vi "PI_12.vi"(7 "SLMAX":fxp<+/-,18,5>, 10 "ziyi_f_in":T1=[0.0, 0.0, 0.0, 0.0, 0.0, 0.0, 0.0, 0.0, 0.0, 0.0, 0.0, 0.0]) -> (2 "ziyi_f_out":T1)   [LabVIEW 2017]
uses:
  ziyi_pipe.ctl
  x_qp_scalar.ctl
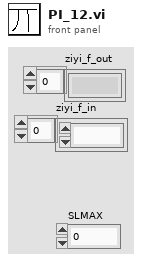
[diagram p1: front panel]
types:
  T1 = typedef "ziyi_pipe.ctl" = T2[]
  T2 = typedef "x_qp_scalar.ctl" = fxp<+/-,32,6>
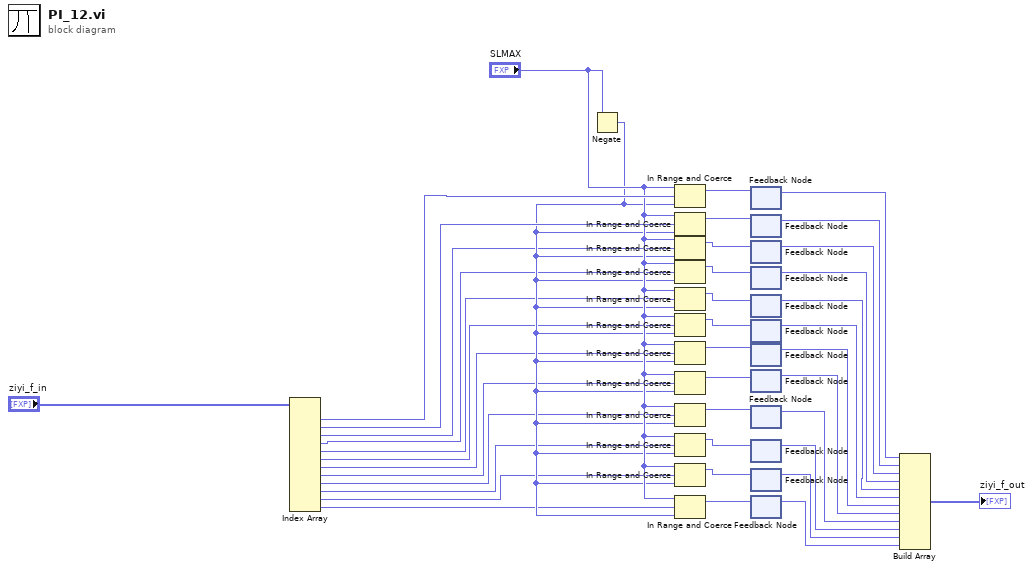
[diagram p0: block diagram]
diagram:
  n1 = Index Array(array="ziyi_f_in") -> (element #1=w16:T2, element #2=w15:T2, element #3=w12:T2, element #4=w11:T2, element #5=w10:T2, element #6=w9:T2, element #7=w8:T2, element #8=w7:T2, element #9=w6:T2, element #10=w5:T2, element #11=w4:T2, element #12=w3:T2)  [unwired: 12 in]
  n2 = Negate(x="SLMAX") -> (-x=w13:fxp<+/-,18,4>)
  n3 = In Range and Coerce(upper limit="SLMAX", x=w16, lower limit=w13) -> (coerced(x)=w40:T2)  [unwired: 1 out]
  n4 = In Range and Coerce(upper limit="SLMAX", x=w15, lower limit=w13) -> (coerced(x)=w39:T2)  [unwired: 1 out]
  n5 = In Range and Coerce(upper limit="SLMAX", x=w12, lower limit=w13) -> (coerced(x)=w38:T2)  [unwired: 1 out]
  n6 = In Range and Coerce(upper limit="SLMAX", x=w11, lower limit=w13) -> (coerced(x)=w37:T2)  [unwired: 1 out]
  n7 = In Range and Coerce(upper limit="SLMAX", x=w10, lower limit=w13) -> (coerced(x)=w36:T2)  [unwired: 1 out]
  n8 = In Range and Coerce(upper limit="SLMAX", x=w9, lower limit=w13) -> (coerced(x)=w35:T2)  [unwired: 1 out]
  n9 = In Range and Coerce(upper limit="SLMAX", x=w8, lower limit=w13) -> (coerced(x)=w34:T2)  [unwired: 1 out]
  n10 = In Range and Coerce(upper limit="SLMAX", x=w7, lower limit=w13) -> (coerced(x)=w33:T2)  [unwired: 1 out]
  n11 = In Range and Coerce(upper limit="SLMAX", x=w6, lower limit=w13) -> (coerced(x)=w32:T2)  [unwired: 1 out]
  n12 = In Range and Coerce(upper limit="SLMAX", x=w5, lower limit=w13) -> (coerced(x)=w31:T2)  [unwired: 1 out]
  n13 = In Range and Coerce(upper limit="SLMAX", x=w4, lower limit=w13) -> (coerced(x)=w30:T2)  [unwired: 1 out]
  n14 = In Range and Coerce(upper limit="SLMAX", x=w3, lower limit=w13) -> (coerced(x)=w29:T2)  [unwired: 1 out]
  n15 = feedback #1() -> (w28:T2)  [unwired: 1 in]
  n16 = feedback-in #1(w40) -> ()
  n17 = feedback #2() -> (w27:T2)  [unwired: 1 in]
  n18 = feedback-in #2(w39) -> ()
  n19 = feedback #3() -> (w26:T2)  [unwired: 1 in]
  n20 = feedback-in #3(w38) -> ()
  n21 = feedback #4() -> (w25:T2)  [unwired: 1 in]
  n22 = feedback-in #4(w37) -> ()
  n23 = feedback #5() -> (w24:T2)  [unwired: 1 in]
  n24 = feedback-in #5(w36) -> ()
  n25 = feedback #6() -> (w23:T2)  [unwired: 1 in]
  n26 = feedback-in #6(w35) -> ()
  n27 = feedback #7() -> (w22:T2)  [unwired: 1 in]
  n28 = feedback-in #7(w34) -> ()
  n29 = feedback #8() -> (w21:T2)  [unwired: 1 in]
  n30 = feedback-in #8(w33) -> ()
  n31 = feedback #9() -> (w20:T2)  [unwired: 1 in]
  n32 = feedback-in #9(w32) -> ()
  n33 = feedback #10() -> (w19:T2)  [unwired: 1 in]
  n34 = feedback-in #10(w31) -> ()
  n35 = feedback #11() -> (w18:T2)  [unwired: 1 in]
  n36 = feedback-in #11(w30) -> ()
  n37 = feedback #12() -> (w17:T2)  [unwired: 1 in]
  n38 = feedback-in #12(w29) -> ()
  n39 = Build Array(w28, w27, w26, w25, w24, w23, w22, w21, w20, w19, w18, w17) -> (→"ziyi_f_out":T2[])
